vi "Main.vi"(10 "Adquisicion":refnum<vi>, 11 "Module Admin":refnum<class "Delacor_lib_QMH_Module Admin.lvclass">) -> ()   [LabVIEW 2019, in "Adquisition.lvlib"]
doc: "This template is based off of the Queued Message Handler design pattern and the Queued Message Handler project template that ships with LabVIEW.\n\nThe main difference is that the queue is private to this module and communication between modules is performed via Broadcast and Request events.\n\nRequest events are wrapped in public API methods and are handled in the Event Handling Loop (EHL) of this VI. Any module can register for Broadcast events sent by this module. The EHL generates messages based on user interface actions.\n\nThe Message Handling Loop (MHL) processes messages generated by the EHL, or by other messages. The messages are string values, so new messages can be added easily to the Message Cases case structure in the MHL. Each message cluster can also provide an optional value for Message Data, which is a variant that can be converted to whatever message-specific data is required.\n_____\nBased on Delacor QMH Project Template 5.0.0.82."
uses:
  Adquisition.lvlib
  <vilib>/Delacor/Delacor QMH/Libraries/Module Admin_class/Delacor_lib_QMH_Module Admin.lvclass
  <vilib>/userdefined/High Color/IMAQdx.ctl
  Module Data--cluster.ctl
  Stop Argument--cluster.ctl
  <vilib>/Delacor/Delacor QMH/Libraries/Message Queue_class/Delacor_lib_QMH_Message Queue.lvclass/Delacor_lib_QMH_Message Queue.ctl
  <vilib>/Delacor/Delacor QMH/Libraries/Module Admin_class/Delacor_lib_QMH_Module Admin.lvclass/Delacor_lib_QMH_Module Admin.ctl
  <vilib>/Utility/miscctls.llb/LVPointTypeDef.ctl
  <vilib>/Delacor/Delacor QMH/Libraries/Message Queue_class/Delacor_lib_QMH_Enqueue Message (Single).vi
  <vilib>/Delacor/Delacor QMH/Libraries/Module Admin_class/Delacor_lib_QMH_Get External Launch.vi
  <vilib>/Utility/error.llb/Error Cluster From Error Code.vi
  <vilib>/ErrorRing/Error Ring.xnode
  <vilib>/Delacor/Delacor QMH/Libraries/Message Queue_class/Delacor_lib_QMH_Message Queue.lvclass
  <vilib>/vision/driver/NI_Vision_Acquisition_Software.lvlib
  Analisis/Analisis.lvlib
panel:
  out "Image Out 2":T1(plugin-control)
  out "error out":errorcluster
  out "Status":string
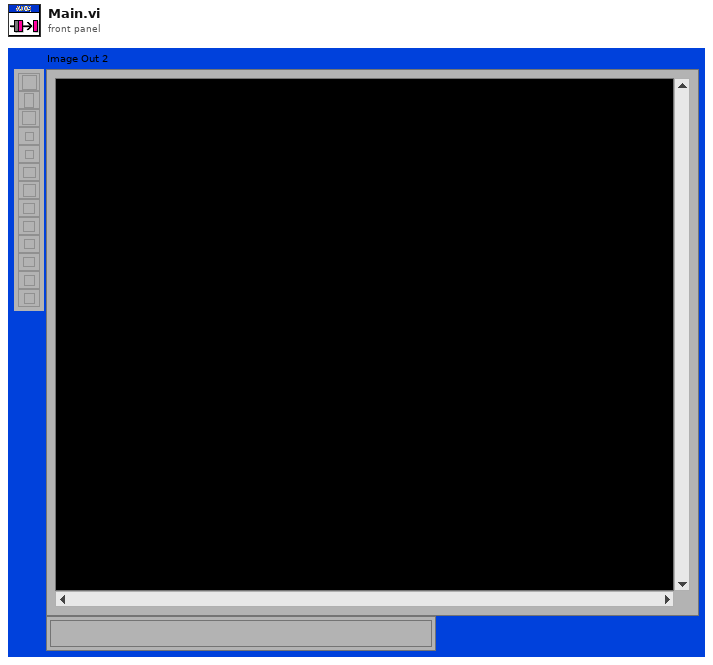
[diagram p1: front panel]
types:
  T1 = typedef "IMAQ Image.ctl" = refnum<image>
  T2 = typedef "IMAQdx.ctl" = refnum<k21>
  T3 = typedef "Adquisition.lvlib/Request Events--cluster.ctl" = cluster{"Stop Module":refnum<user-event>, "Show Panel":refnum<user-event>, "Hide Panel":refnum<user-event>, "Get Module Execution Status":refnum<user-event>, "Show Diagram":refnum<user-event>, "start adquisition":refnum<user-event>, "stop adquisition":refnum<user-event>, "color selection":refnum<user-event>}
  T4 = typedef "Adquisition.lvlib/Module Data--cluster.ctl" = cluster{"Status":string}
  T5 = enum32{"invalid lock state", "Not Locked", "Locked (No Password)", "Password-protected"}
  T6 = typedef "Adquisition.lvlib/Stop Argument--cluster.ctl" = cluster{"Origin":string, "Exit via Stop Module Req?":bool, "Wait for Module to stop?":bool}
  T7 = typedef "LVPointTypeDef.ctl" = cluster{"Horizontal":i16, "Vertical":i16}
  T8 = enum32{"Invalid", "Standard", "Closed", "Hidden", "Minimized", "Maximized"}
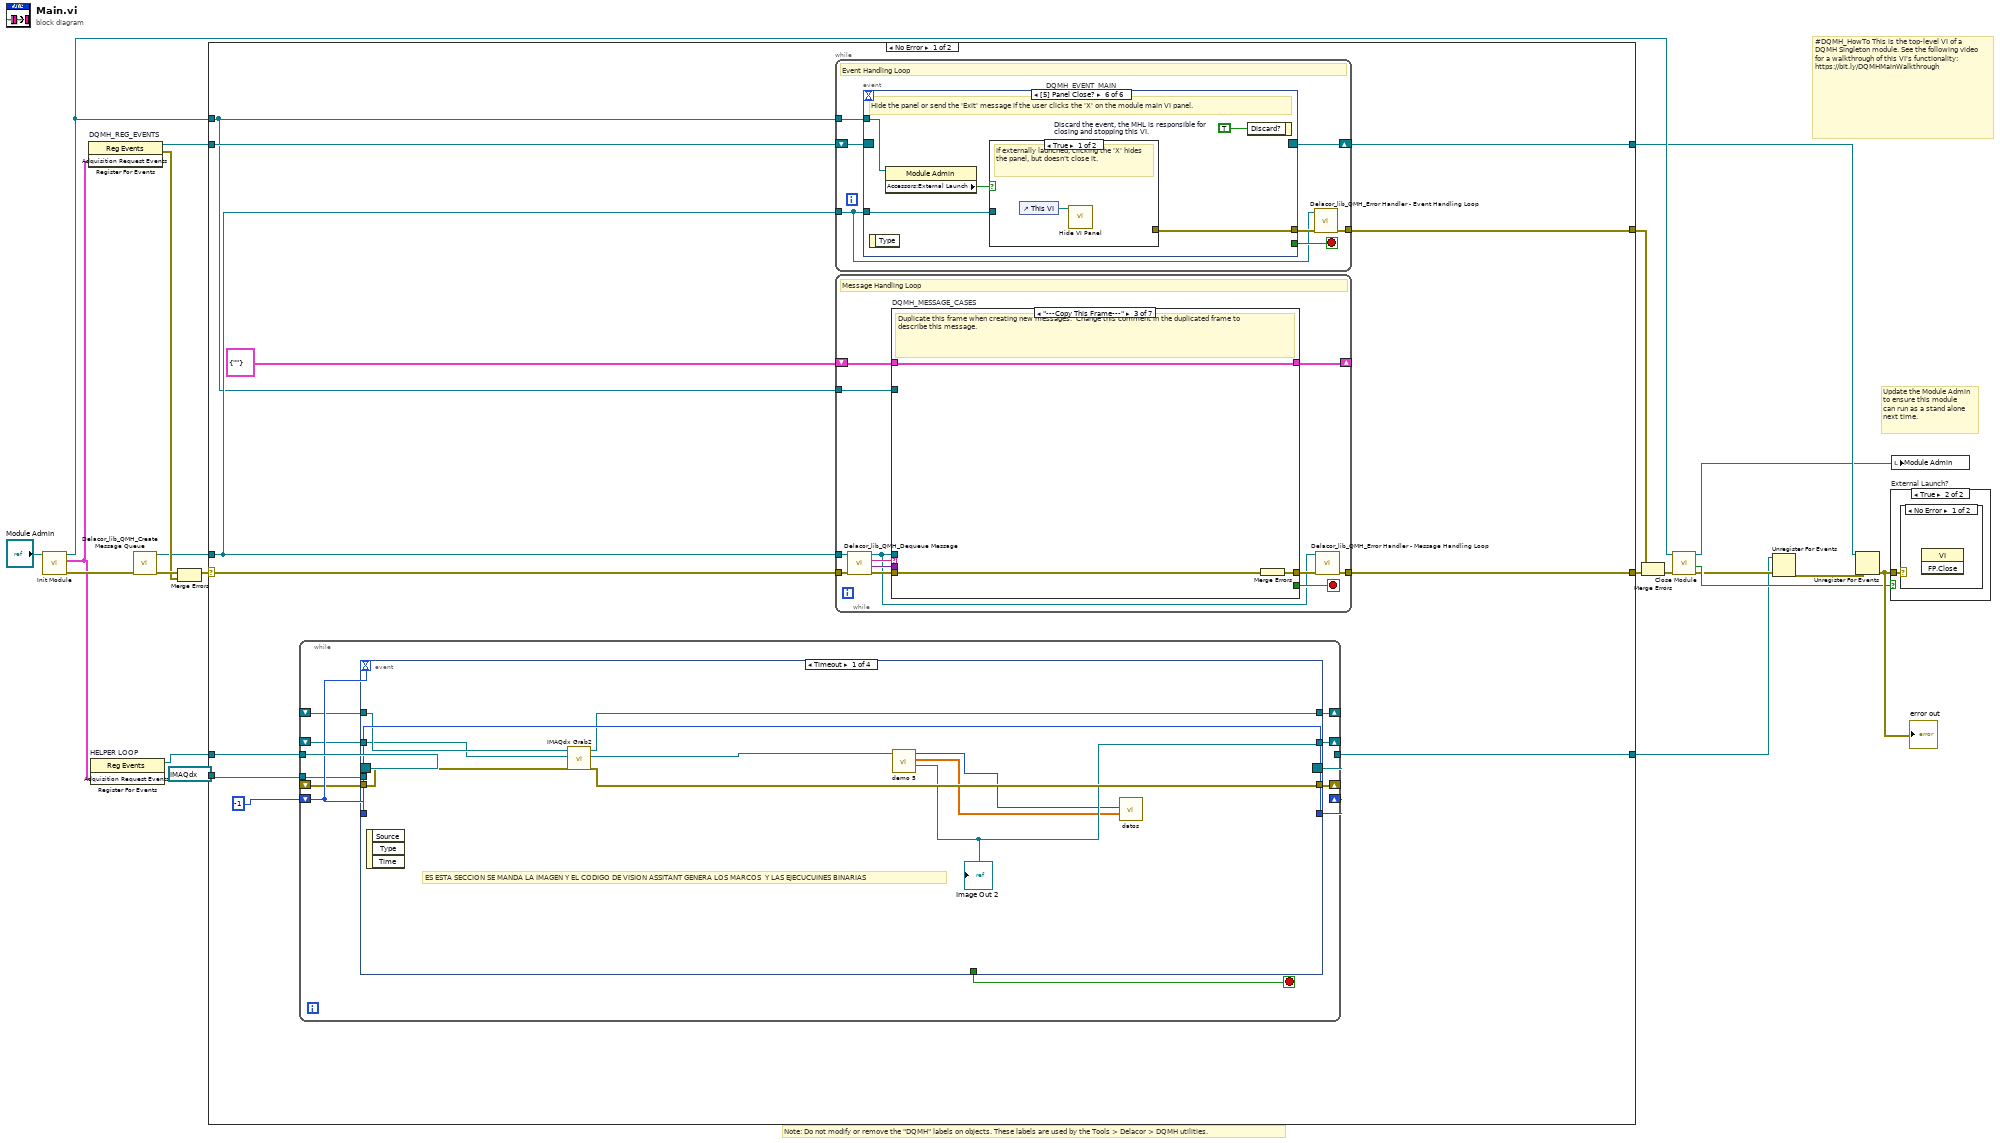
[diagram p0: block diagram]
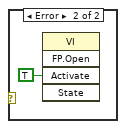
[diagram p3: hidden frame]
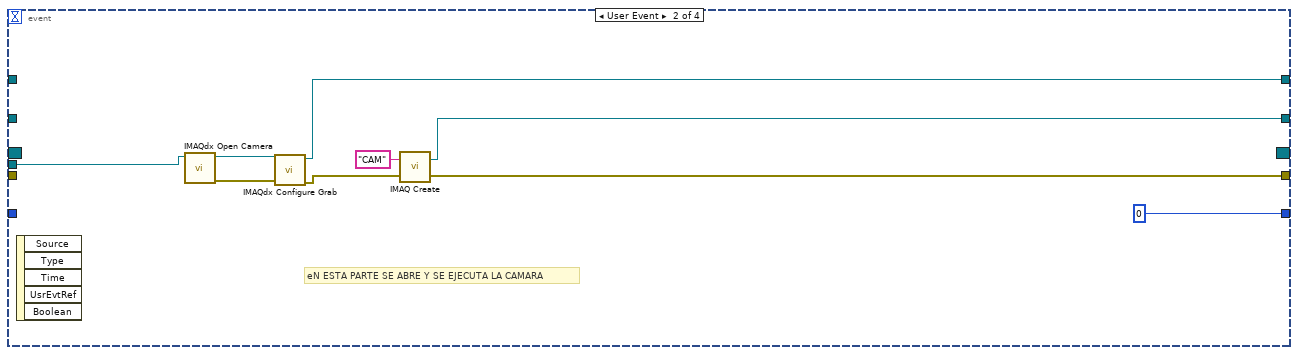
[diagram p4: hidden frame]
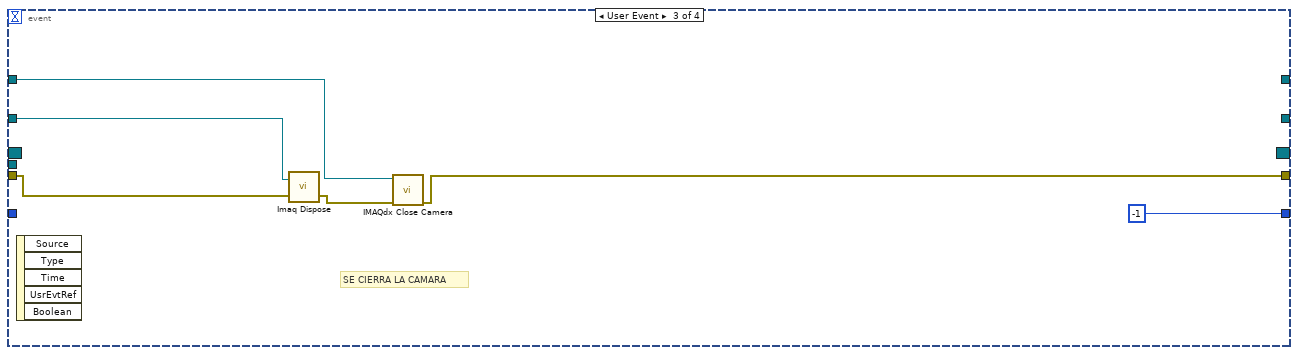
[diagram p5: hidden frame]
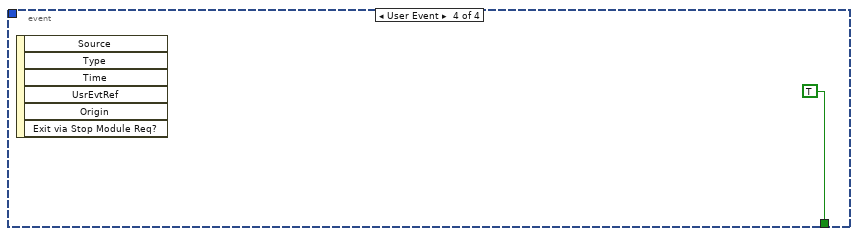
[diagram p6: hidden frame]
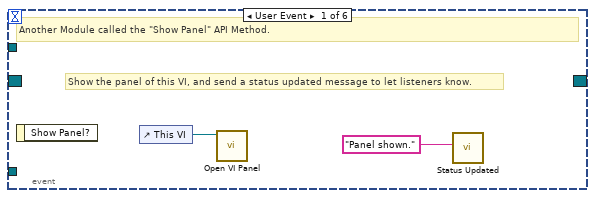
[diagram p7: hidden frame]
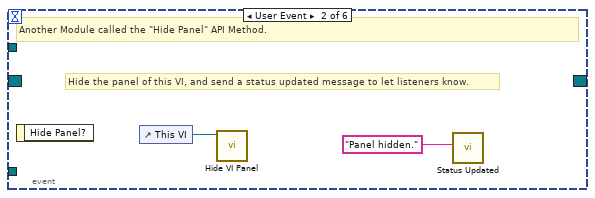
[diagram p8: hidden frame]
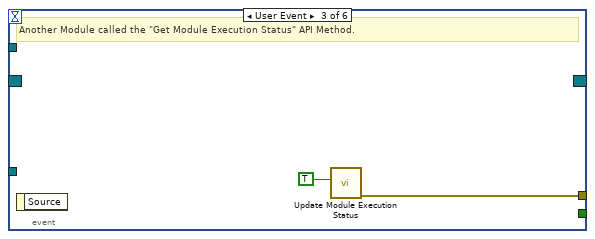
[diagram p9: hidden frame]
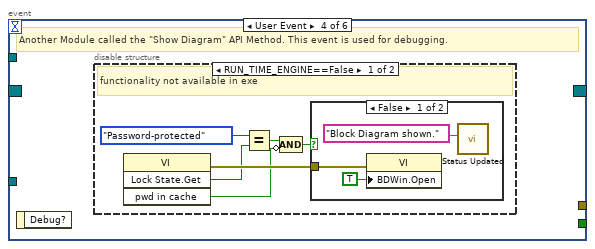
[diagram p10: hidden frame]
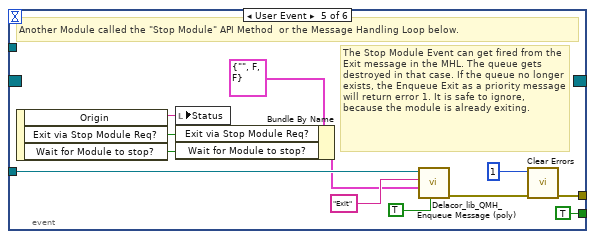
[diagram p13: hidden frame]
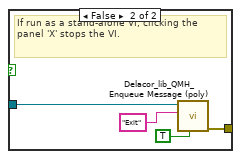
[diagram p14: hidden frame]
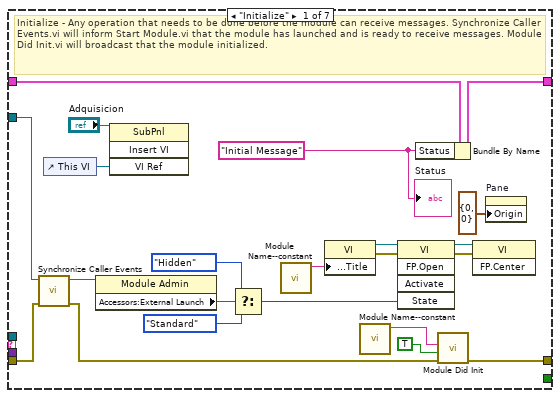
[diagram p15: hidden frame]
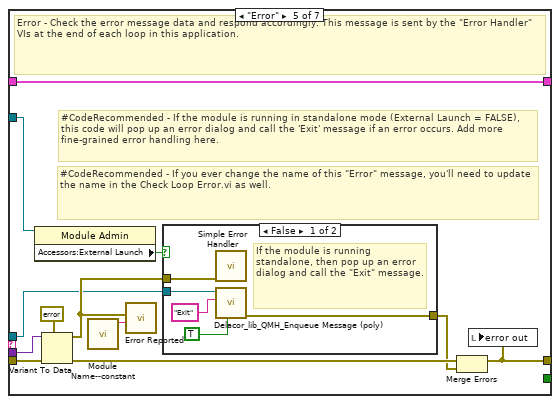
[diagram p18: hidden frame]
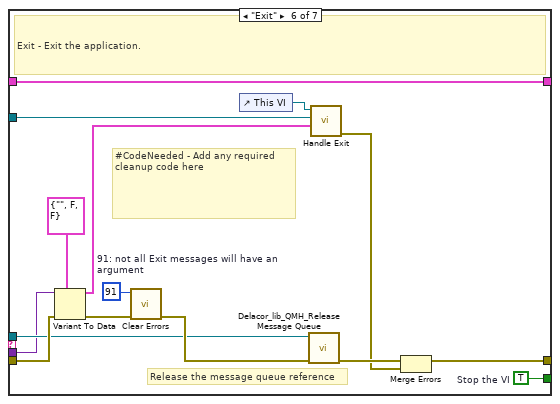
[diagram p20: hidden frame]
diagram:
  # "#DQMH_HowTo This is the top-level VI of a DQMH Singleton module. See the following video for a walkthrough of this VI's functionality: https://bit.ly/DQMHMainWalkthrough"
  # "Note: Do not modify or remove the \"DQMH\" labels on objects. These labels are used by the Tools > Delacor > DQMH utilities."
  # "Update the Module Admin to ensure this module can run as a stand alone next time."
  n1 = call "Init Module.vi"("Singleton Module Admin in"="Module Admin") -> ("error out"=w20:errorcluster, "Adquisition Request Events"=w6:T3, "Singleton Module Admin out"=w13:refnum<class "Delacor_lib_QMH_Module Admin.lvclass">)  [unwired: 8 in]
  n2 = register-events "DQMH_REG_EVENTS"(w6) -> (reference out=w11:refnum<event-registration>, error out=w14:errorcluster)  [unwired: 2 in]
  n3 = register-events "HELPER LOOP"(w6) -> (reference out=w5:refnum<event-registration>)  [unwired: 2 in, 1 out]
  n4 = call <vilib>:"Delacor_lib_QMH_Create Message Queue.vi"("error in (no error)"=w20) -> ("error out"=w16:errorcluster, "Message Queue"=w10:refnum<class "Delacor_lib_QMH_Message Queue.lvclass">)  [unwired: 9 in]
  n5 = Merge Errors(w16, w14) -> (w15:errorcluster)
  n6 = case shown="No Error" w15 {
    selector: w15 -> [w31 w206]
    tunnel: [w33 w205] -> w21
    tunnel: [w30 w211] -> w12
    tunnel: w11 -> [w28 w211]
    tunnel: w10 -> [w27 w204]
    tunnel: [w32 _] -> w19
    tunnel: w13 -> [w26 w207]
    tunnel: w5 -> [w25 w203]
    tunnel: [w24 w203] -> w2
    tunnel: T2 "cam1" ("Session In") -> [w22 _]
    frame No Error {
      n7 = while {
        tunnel: w25 -> [w45]
        tunnel: [w44] -> w24
        shift-right: [w42] -> _
        shift-left: -1 -> [w43]
        tunnel: w22 -> [w40]
        shift-right: [w39] -> _
        shift-left: _ -> [w35]
        shift-right: [w37] -> _
        shift-left: _ -> [w36]
        shift-right: [w38] -> _
        shift-left: _ -> [w34]
        stop <- w41 stop-if-true
        n8 = event shown="[0] Timeout" {
          selector: w45 -> [_ _ _ _]
          dyn-events: [_ _ _ _] -> w44
          timeout: w43 -> [_ _ _ _]
          tunnel: w43 -> [w55 _ _ _]
          tunnel: [w55 0 -1 _] -> w42
          tunnel: [_ _ _ TRUE] -> w41
          tunnel: w40 -> [_ w63 _ _]
          tunnel: [w51 w60 _ _] -> w39
          tunnel: [w50 w58 w65 _] -> w38
          tunnel: [w48 w57 _ _] -> w37
          tunnel: w36 -> [w52 _ w69 _]
          tunnel: w35 -> [w53 _ w68 _]
          tunnel: w34 -> [w54 _ w67 _]
          event Timeout {
            # "ES ESTA SECCION SE MANDA LA IMAGEN Y EL CODIGO DE VISION ASSITANT GENERA LOS MARCOS  Y LAS EJECUCUINES BINARIAS"
            n9 = event-data() -> ()  [unwired: 1 in, 3 out]
            n10 = call <vilib>:"IMAQdx Grab2.vi"("error in"=w54, "Image In"=w52, "Session In"=w53) -> ("error out"=w50:errorcluster, "Image Out"=w49:T1, "Session Out"=w51:T2)  [unwired: 5 in, 1 out]
            n11 = call "demo 5.vi"("Image Src"=w49) -> ("Image Out"=w48:T1, "Particle Measurements (Pixels) (Particle Analysis 1)"=w46:dbl[][], "Number of Particles (Particle Analysis 1)"=w47:i32)  [unwired: 5 in, 1 out]
            "Image Out 2" <- w48
            n12 = call "datos.vi"("Particle Measurements (Pixels) (Particle Analysis 1)"=w46, "Numero de monedas"=w47) -> ()  [unwired: 9 in, 1 out]
          }
          event User Event {
            # "eN ESTA PARTE SE ABRE Y SE EJECUTA LA CAMARA"
            n13 = event-data() -> ()  [unwired: 1 in, 5 out]
            n14 = call <vilib>:"IMAQdx Open Camera.vi"("Session In"=w63) -> ("error out"=w61:errorcluster, "Session Out"=w62:T2)  [unwired: 9 in]
            n15 = call <vilib>:"IMAQdx Configure Grab.vi"("error in"=w61, "Session In"=w62) -> ("error out"=w59:errorcluster, "Session Out"=w60:T2)  [unwired: 8 in]
            n16 = call "IMAQ Create"("Image Name"="CAM", "error in (no error)"=w59) -> ("New Image"=w57:T1, "error out"=w58:errorcluster)  [unwired: 3 in]
          }
          event User Event {
            # "SE CIERRA LA CAMARA"
            n17 = event-data() -> ()  [unwired: 1 in, 5 out]
            n18 = call "Imaq Dispose"("Image"=w69, "error in (no error)"=w67) -> ("error out"=w66:errorcluster)  [unwired: 4 in]
            n19 = call <vilib>:"IMAQdx Close Camera.vi"("error in"=w66, "Session In"=w68) -> ("error out"=w65:errorcluster)  [unwired: 9 in]
          }
          event User Event {
            n20 = event-data() -> ()  [unwired: 1 in, 6 out]
          }
        }
      }
      n21 = while {
        tunnel: w27 -> [w72]
        shift-right: [w75] -> w30
        shift-left: w28 -> [w76]
        tunnel: [w77] -> w32
        tunnel: w26 -> [w73]
        stop <- w74 stop-if-true
        # "Event Handling Loop"
        n22 = event "DQMH_EVENT_MAIN" shown="[5] Panel Close?" {
          selector: w76 -> [_ _ _ _ _ _]
          dyn-events: [_ _ _ _ _ _] -> w75
          timeout: _ -> [_ _ _ _ _ _]
          tunnel: [_ _ _ _ TRUE ("Discard?") _] -> w74
          tunnel: w72 -> [_ _ _ _ w101 w108]
          tunnel: [_ _ w84 _ w104 w110] -> w78
          tunnel: w73 -> [_ _ _ _ _ w107]
          event User Event {
            # "Show the panel of this VI, and send a status updated message to let listeners know."
            # "Another Module called the \"Show Panel\" API Method."
            n23 = event-data() -> ()  [unwired: 1 in, 1 out]
            n24 = control-ref of="This VI"() -> (w80:refnum<vi>)
            n25 = call "Open VI Panel.vi"("VI"=w80) -> ()  [unwired: 10 in, 1 out]
            n26 = call "Status Updated.vi"("Status"="Panel shown." ("format string")) -> ()  [unwired: 10 in, 1 out]
          }
          event User Event {
            # "Hide the panel of this VI, and send a status updated message to let listeners know."
            # "Another Module called the \"Hide Panel\" API Method."
            n27 = event-data() -> ()  [unwired: 1 in, 1 out]
            n28 = control-ref of="This VI"() -> (w82:refnum<vi>)
            n29 = call "Hide VI Panel.vi"("VI"=w82) -> ()  [unwired: 10 in, 1 out]
            n30 = call "Status Updated.vi"("Status"="Panel hidden." ("format string")) -> ()  [unwired: 10 in, 1 out]
          }
          event User Event {
            # "Another Module called the \"Get Module Execution Status\" API Method."
            n31 = event-data() -> ()  [unwired: 1 in, 1 out]
            n32 = call "Update Module Execution Status.vi"("Running?"=TRUE) -> ("error out"=w84:errorcluster)  [unwired: 10 in]
          }
          event User Event {
            # "Another Module called the \"Show Diagram\" API Method. This event is used for debugging."
            n33 = event-data() -> ()  [unwired: 1 in, 1 out]
            n34 = disable-structure shown="RUN_TIME_ENGINE==False" {
              frame condition #0 (active) {
                # "functionality not available in exe"
                n35 = invoke class="VI" method="Lock State.Get"() -> (error out=w90:errorcluster, "Get Lock State"=w89:T5, "pwd in cache"=w86:bool)  [unwired: 4 in, 1 out]
                n36 = Equal?(x=T5."Password-protected", y=w89) -> (x = y?=w87:bool)
                n37 = Compound Arithmetic op=AND(w87, invert w86) -> (w85:bool)
                n38 = case shown="False" w85 {
                  tunnel: w90 -> [w93 _]
                  frame False {
                    n39 = property class="VI"(error in=w93, "BDWin.Open"=TRUE ("Block Diagram Window:Open")) -> ()  [unwired: 1 in, 2 out]
                    n40 = call "Status Updated.vi"("Status"="Block Diagram shown." ("format string")) -> ()  [unwired: 10 in, 1 out]
                  }
                  frame True {
                    # "Password-protected VI, and the password is not in the cache. Do not show the diagram."
                  }
                }
              }
              frame condition #1 {
              }
            }
          }
          event User Event {
            # "The Stop Module Event can get fired from the Exit message in the MHL. The queue gets destroyed in that case. If the queue no longer exists, the Enqueue Exit as a priority message will return error 1. It is safe to ignore, because the module is already exiting."
            # "Another Module called the \"Stop Module\" API Method  or the Message Handling Loop below."
            n41 = event-data() -> ("Origin"=w100:string, "Exit via Stop Module Req?"=w96:bool, "Wait for Module to stop?"=w95:bool)  [unwired: 1 in]
            n42 = local write "Status"(w100) -> ()
            n43 = Bundle By Name(cluster=T6 {"Origin"="", "Exit via Stop Module Req?"=FALSE, "Wait for Module to stop?"=FALSE} ("Stop Argument"), "Exit via Stop Module Req?"=w96, "Wait for Module to stop?"=w95) -> (w94:T6)
            n44 = call-poly <vilib>:"Delacor_lib_QMH_Enqueue Message (poly).vi"("Priority Message? (F)"=TRUE, "Message Data"=w94, "Message"="Exit", "Message Queue in"=w101) -> ("error out"=w105:errorcluster)  [unwired: 6 in, 1 out]
            n45 = call <vilib>:"Clear Errors.vi"("error in (no error)"=w105, "specific error code to clear (0: all)"=1) -> ("error out"=w104:errorcluster)  [unwired: 4 in, 1 out]
          }
          event Panel Close? {
            w109 = TRUE  # Discard the event, the MHL is responsible for closing and stopping this VI.
            # "Hide the panel or send the 'Exit' message if the user clicks the 'X' on the module main VI panel."
            n46 = event-data() -> ()  [unwired: 1 in, 1 out]
            n47 = property class="Module Admin"(reference=w107) -> ("Accessors:External Launch"=w106:bool)  [unwired: 1 in, 2 out]
            n48 = case shown="True" w106 {
              tunnel: w108 -> [_ w114]
              tunnel: [_ w115] -> w110
              frame True {
                # "If externally launched, clicking the 'X' hides the panel, but doesn't close it."
                n49 = control-ref of="This VI"() -> (w111:refnum<vi>)
                n50 = call "Hide VI Panel.vi"("VI"=w111) -> ()  [unwired: 10 in, 1 out]
              }
              frame False {
                # "If run as a stand-alone VI, clicking the panel 'X' stops the VI."
                n51 = call-poly <vilib>:"Delacor_lib_QMH_Enqueue Message (poly).vi"("Priority Message? (F)"=TRUE, "Message"="Exit", "Message Queue in"=w114) -> ("error out"=w115:errorcluster)  [unwired: 7 in, 1 out]
              }
            }
            n52 = event-data("Discard?"=w109) -> ()  [unwired: 1 in, 1 out]
          }
        }
        n53 = call-dynamic "Delacor_lib_QMH_Error Handler - Event Handling Loop.vi"("error in (no error)"=w78, "Message Queue in"=w72) -> ("dup error in"=w77:errorcluster)  [unwired: 8 in, 1 out]
      }
      n54 = while {
        tunnel: w27 -> [w118]
        shift-right: [w122] -> _
        shift-left: T4 {"Status"=""} ("Data Cluster") -> [w123]
        tunnel: w31 -> [w126]
        tunnel: [w124] -> w33
        tunnel: w26 -> [w116]
        stop <- w121 stop-if-true
        # "Message Handling Loop"
        n55 = call-dynamic "Delacor_lib_QMH_Dequeue Message.vi"("error in (no error)"=w126, "Message Queue in"=w118) -> ("error out"=w125:errorcluster, "Message Data"=w119:variant, "Message"=w120:string, "Message Queue out"=w117:refnum<class "Delacor_lib_QMH_Message Queue.lvclass">)  [unwired: 6 in]
        n56 = case "DQMH_MESSAGE_CASES" shown="\"---Copy This Frame---\"" w120 {
          selector: w120 -> [_ _ _ _ _ _ w190]
          tunnel: w117 -> [_ _ _ _ w160 w182 _]
          tunnel: w125 -> [w147 w151 w154 w156 w167 w188 w192]
          tunnel: [w145 w151 w153 w156 w163 w185 w193] -> w127
          tunnel: w123 -> [w136 w150 w152 w155 w162 w181 w191]
          tunnel: [w135 w150 w152 w155 w162 w181 w191] -> w122
          tunnel: [_ _ _ _ _ w180 _] -> w121
          tunnel: w119 -> [_ _ _ _ w161 w179 _]
          tunnel: w116 -> [w137 _ _ _ w159 w174 _]
          frame "Initialize" {
            w130 = "Initial Message" ("Initial Message")
            # "Initialize - Any operation that needs to be done before the module can receive messages. Synchronize Caller Events.vi will inform Start Module.vi that the module has launched and is ready to receive messages. Module Did Init.vi will broadcast that the module initialized."
            n57 = call "Synchronize Caller Events.vi"("error in (no error)"=w147, "Singleton Module Admin in"=w137) -> ("error out"=w146:errorcluster, "Singleton Module Admin out"=w132:refnum<class "Delacor_lib_QMH_Module Admin.lvclass">)  [unwired: 8 in]
            n58 = control-ref of="This VI"() -> (w128:refnum<vi>)
            n59 = property class="Module Admin"(reference=w132) -> ("Accessors:External Launch"=w141:bool)  [unwired: 1 in, 2 out]
            n60 = invoke class="SubPnl" method="Insert VI"(reference="Adquisicion", "VI Ref"=w128) -> ()  [unwired: 2 in, 4 out]
            n61 = Select(t=T8."Hidden" ("State"), s=w141, f=T8."Standard" ("State")) -> (s? t:f=w138:T8)
            n62 = call "Module Name--constant.vi"() -> ("Module Name"=w144:string)  [unwired: 11 in]
            n63 = property class="VI"("Front Panel.Title"=w144) -> (reference out=w143:refnum<vi>, error out=w149:errorcluster)  [unwired: 2 in]
            n64 = call "Module Name--constant.vi"() -> ("Module Name"=w133:string)  [unwired: 11 in]
            n65 = invoke class="VI" method="FP.Open"(reference=w143, error in=w149, "State"=w138) -> (reference out=w142:refnum<vi>, error out=w148:errorcluster)  [unwired: 2 in, 3 out]
            n66 = Bundle By Name(cluster=w136, "Status"=w130) -> (w135:T4)
            n67 = call "Module Did Init.vi"("error in (no error)"=w146, "Initialized?"=TRUE, "Origin"=w133) -> ("error out"=w145:errorcluster)  [unwired: 8 in]
            n68 = invoke class="VI" method="FP.Center"(reference=w142, error in=w148) -> ()  [unwired: 1 in, 3 out]
            n69 = property on="Pane" class="Pane"("Origin"=T7 {"Horizontal"=0, "Vertical"=0}) -> ()  [unwired: 2 in, 2 out]
            "Status" <- w130
          }
          frame "--- Module Specific ---" {
            # "Separator -- The following cases handle messages specific to this Module."
          }
          frame "---Copy This Frame---" {
            # "Duplicate this frame when creating new messages.  Change this comment in the duplicated frame to describe this message."
            n70 = Merge Errors(w154) -> (w153:errorcluster)
          }
          frame "--- Exit and Error Handling---" {
            # "Separator - The following cases handle errors and exit messages."
          }
          frame "Error" {
            # "#CodeRecommended - If you ever change the name of this \"Error\" message, you'll need to update the name in the Check Loop Error.vi as well."
            # "#CodeRecommended - If the module is running in standalone mode (External Launch = FALSE), this code will pop up an error dialog and call the 'Exit' message if an error occurs. Add more fine-grained error handling here."
            # "Error - Check the error message data and respond accordingly. This message is sent by the \"Error Handler\" VIs at the end of each loop in this application."
            n71 = property class="Module Admin"(reference=w159) -> ("Accessors:External Launch"=w158:bool)  [unwired: 1 in, 2 out]
            n72 = Variant To Data(error in=w167, type=errorcluster {"status"=FALSE, "code"=0, "source"=""} ("error constant"), Variant=w161) -> (data=w168:errorcluster, error out=w165:errorcluster)
            n73 = call "Module Name--constant.vi"() -> ("Module Name"=w157:string)  [unwired: 11 in]
            n74 = call "Error Reported.vi"("Additional Information"=w157, "Error"=w168) -> ()  [unwired: 9 in, 1 out]
            n75 = case shown="False" w158 {
              tunnel: [w173 _] -> w164
              tunnel: w160 -> [w171 _]
              tunnel: w168 -> [w172 _]
              frame False {
                # "If the module is running standalone, then pop up an error dialog and call the \"Exit\" message."
                n76 = call <vilib>:"Simple Error Handler.vi"("error in (no error)"=w172) -> ()  [unwired: 4 in, 5 out]
                n77 = call-poly <vilib>:"Delacor_lib_QMH_Enqueue Message (poly).vi"("Priority Message? (F)"=TRUE, "Message"="Exit", "Message Queue in"=w171) -> ("error out"=w173:errorcluster)  [unwired: 7 in, 1 out]
              }
              frame True {
                # "If the module was launched externally, calling the Error Reported broadcast VI is the only action performed by the \"Error\" message. The module's caller can then process the error appropriately."
              }
            }
            n78 = Merge Errors(w165, w164) -> (w163:errorcluster)
            n79 = local write "error out"(w163) -> ()
          }
          frame "Exit" {
            w178 = 91  # 91: not all Exit messages will have an argument
            w180 = TRUE  # Stop the VI
            # "Release the message queue reference"
            # "#CodeNeeded - Add any required cleanup code here"
            # "Exit - Exit the application."
            n80 = Variant To Data(error in=w188, type=T6 {"Origin"="", "Exit via Stop Module Req?"=FALSE, "Wait for Module to stop?"=FALSE} ("Stop Argument"), Variant=w179) -> (data=w176:T6, error out=w184:errorcluster)
            n81 = call <vilib>:"Clear Errors.vi"("error in (no error)"=w184, "specific error code to clear (0: all)"=w178) -> ("error out"=w187:errorcluster)  [unwired: 4 in, 1 out]
            n82 = control-ref of="This VI"() -> (w175:refnum<vi>)
            n83 = call-dynamic "Delacor_lib_QMH_Release Message Queue.vi"("error in (no error)"=w187, "Message Queue"=w182) -> ("error out"=w186:errorcluster)  [unwired: 9 in]
            n84 = call "Handle Exit.vi"("Stop Argument"=w176, "Admin in"=w174, "VI reference"=w175) -> ("error out"=w183:errorcluster)  [unwired: 7 in, 1 out]
            n85 = Merge Errors(w186, w183) -> (w185:errorcluster)
          }
          frame Default {
            # "'Default' case only runs if there is a message that isn't defined in any of the other cases.  Output a programming error."
            n86 = call "Module Name--constant.vi"() -> ("Module Name"=w189:string)  [unwired: 11 in]
            n87 = xnode "Error Ring"("parameter 0"=w190, "parameter 1"=w189) -> ("error out"=w194:errorcluster)
            n88 = Merge Errors(w192, w194) -> (w193:errorcluster)
          }
        }
        n89 = call-dynamic "Delacor_lib_QMH_Error Handler - Message Handling Loop.vi"("error in (no error)"=w127, "Message Queue in"=w117) -> ("dup error in"=w124:errorcluster)  [unwired: 8 in, 1 out]
      }
    }
    frame Error {
      # "Synchronize Caller Events.vi will inform Start Module.vi that the module has launched and will let the code calling Start Module.vi register for broadcasts and would permit the caller receive the broadcast that an error occurred at launch time."
      n90 = call-dynamic "Delacor_lib_QMH_Release Message Queue.vi"("error in (no error)"=w206, "Message Queue"=w204) -> ("error out"=w205:errorcluster)  [unwired: 9 in]
      n91 = call "Synchronize Caller Events.vi"("Singleton Module Admin in"=w207) -> ("error out"=w212:errorcluster)  [unwired: 9 in, 1 out]
      n92 = call "Module Name--constant.vi"() -> ("Module Name"=w210:string)  [unwired: 11 in]
      n93 = Format Into String(format string="An error occurred during initialization. %s is no longer running.", w210) -> (resulting string=w208:string)  [unwired: 2 in, 1 out]
      n94 = Merge Errors(w205, w212) -> (w213:errorcluster)
      n95 = call "Error Reported.vi"("Additional Information"=w208, "Error"=w213) -> ()  [unwired: 9 in, 1 out]
    }
  }
  n96 = Merge Errors(w19, w21) -> (w18:errorcluster)
  n97 = call "Close Module.vi"("error in (no error)"=w18, "Module Admin in"=w13) -> ("error out"=w4:errorcluster, "External Launch"=w7:bool, "Module Admin out"=w8:refnum<class "Delacor_lib_QMH_Module Admin.lvclass">)  [unwired: 7 in]
  n98 = Unregister For Events(event registration refnum=w2, error in=w4) -> (error out=w3:errorcluster)
  n99 = Unregister For Events(event registration refnum=w12, error in=w3) -> (error out=w17:errorcluster)
  "error out" <- w17
  n100 = case "External Launch?" shown="True" w7 {
    tunnel: w17 -> [_ w214]
    frame False {
    }
    frame True {
      n101 = case shown="No Error" w214 {
        frame No Error {
          n102 = invoke class="VI" method="FP.Close"() -> ()  [unwired: 3 in, 3 out]
        }
        frame Error {
          n103 = invoke class="VI" method="FP.Open"("Activate"=TRUE ("Activate?")) -> ()  [unwired: 4 in, 5 out]
        }
      }
    }
  }
  n104 = local write "Module Admin"(w8) -> ()
